vi "Equipos.vi"(2 "error in (no error)":errorcluster, 3 "stop":bool, 4 "Cantidad de alumnos":u32=2 min=2) -> (0 "error out":errorcluster, 1 "Resultado":string caption="Result")   [LabVIEW 2016]
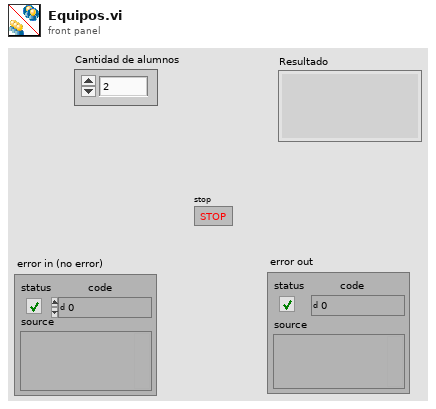
[diagram p1: front panel]
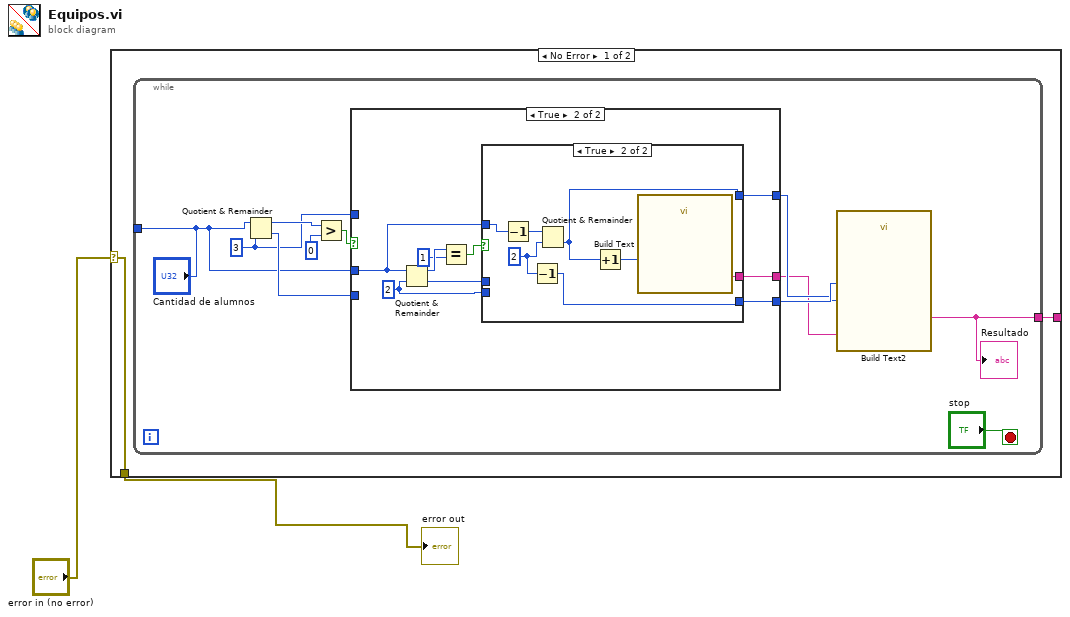
[diagram p0: block diagram]
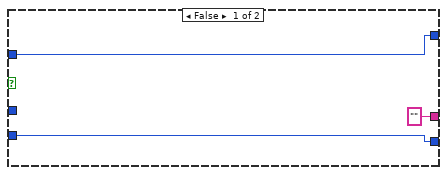
[diagram p2: hidden frame]
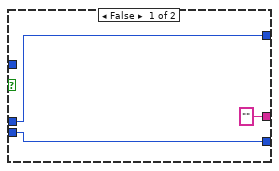
[diagram p3: hidden frame]
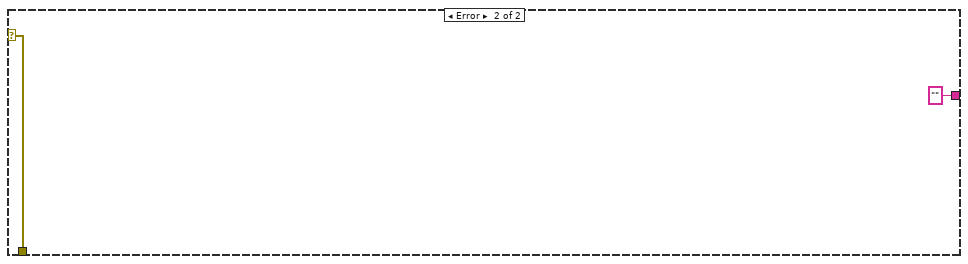
[diagram p4: hidden frame]
diagram:
  n1 = case shown="No Error" "error in (no error)" {
    selector: "error in (no error)" -> [w4 w38]
    tunnel: [w4 w38] -> w1
    tunnel: [w3 "" ("Result")] -> _
    frame No Error {
      n2 = while {
        tunnel: ["Cantidad de alumnos"] -> _
        tunnel: [w5] -> w3
        stop <- "stop" stop-if-true
        w11 = u32 3 ("y")
        n3 = Quotient & Remainder(x="Cantidad de alumnos", y=w11) -> (x-y*floor(x/y)=w13:u32, floor(x/y)=w12:u32)
        n4 = Greater?(x=w13, y=u32 0) -> (0:w14:bool)
        n5 = case shown="True" w14 {
          tunnel: w12 -> [w16 _]
          tunnel: "Cantidad de alumnos" -> [_ w22]
          tunnel: w11 -> [w17 _]
          tunnel: [w16 w21] -> w10
          tunnel: ["" ("Result") w20] -> w8
          tunnel: [w17 w19] -> w9
          frame False {
          }
          frame True {
            w27 = u32 2 ("y")
            n6 = Quotient & Remainder(x=w22, y=w27) -> (x-y*floor(x/y)=w25:u32, floor(x/y)=w26:u32)
            n7 = Equal?(x=w25, y=u32 1) -> (x = y?=w23:bool)
            n8 = case shown="True" w23 {
              tunnel: w27 -> [w29 _]
              tunnel: w26 -> [w30 _]
              tunnel: w22 -> [_ w37]
              tunnel: [w29 w34] -> w21
              tunnel: [w30 w31] -> w19
              tunnel: ["" ("Result") w32] -> w20
              frame False {
              }
              frame True {
                w35 = u32 2 ("y")
                n9 = Decrement(x=w37) -> (x-1=w36:u32)
                n10 = Decrement(x=w35) -> (x-1=w34:u32)
                n11 = Quotient & Remainder(x=w36, y=w35) -> (floor(x/y)=w31:u32)  [unwired: 1 out]
                n12 = Increment(x=w31) -> (x+1=w33:u32)
                n13 = call "Build Text"("IMPAR"=w33) -> ("Result"=w32:string)  [unwired: 13 in, 1 out]
              }
            }
          }
        }
        n14 = call "Build Text2"("EQUIPOS"=w10, "INTEGRANTES"=w9, "NOPAR"=w8) -> ("Result"=w5:string)  [unwired: 11 in, 1 out]
        "Resultado" <- w5
      }
    }
    frame Error {
    }
  }
  "error out" <- w1
